vi "GetDriverName.vi"(8 "Error In":errorcluster, 11 "reference in":refnum<class "VdAnalogInput_DAQmx.lvclass">) -> (0 "Error Out":errorcluster, 2 "DriverName":string, 3 "reference out":refnum<class "VdAnalogInput_DAQmx.lvclass">)   [LabVIEW 2020, in "VdAnalogInput_DAQmx.lvclass"]
uses:
  VdAnalogInput_DAQmx.lvclass
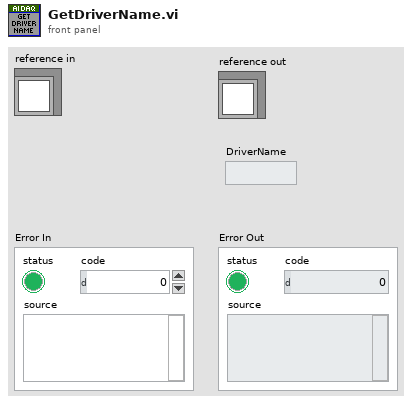
[diagram p1: front panel]
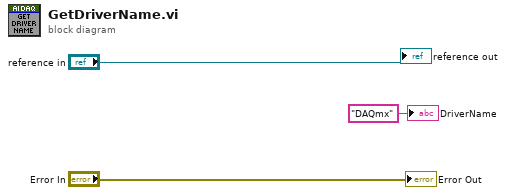
[diagram p0: block diagram]
diagram:
  "Error Out" <- "Error In"
  "reference out" <- "reference in"
  "DriverName" <- "DAQmx" ("DriverName")
